vi "HFRR ADV v04 new software.vi"() -> ()   [LabVIEW 2025] (continued)
            n2731 = Search and Replace String(input string=w3755, search string=".duf", replace string=".dgf" ("replace string (\"\")")) -> (result string=→"String Indicator 4":string)  [unwired: 5 in, 3 out]
            n2732 = Match Pattern(string=w3770, regular expression=".dwm") -> (before substring=w3754:string)  [unwired: 1 in, 3 out]
            "String Indicator" <- w3754
            n2733 = Match Pattern(string=w3755, regular expression=".dwm" ("substring (\"\")")) -> (before substring=w3756:string)  [unwired: 1 in, 3 out]
            "String Indicator 3" <- w3756
            n2734 = local write "TITTLE 2"(w3754) -> ()
            n2735 = String To Path(string=w3756) -> (path=w3763:path)
            "path" <- w3763
            n2736 = call <vilib>:"Read Characters From File.vi"("file path (dialog if empty)"=w3763, "start of read offset (chars.:0)"=60 ("start of read offset (chars.: 0)")) -> ("character string"=→"String Indicator 2":string)  [unwired: 4 in, 3 out]
          }
        }
        n2737 = call <vilib>:"Query Available Printers.vi"() -> ("system configured printers"=w3455:string[])  [unwired: 9 in, 2 out]
        "System Configured Printers 2" <- w3455
        n2738 = local read "OK Button 16"() -> (w3452:bool)
        n2739 = case shown="True" "OK Button 16" {
          frame False {
          }
          frame True {
            n2740 = stacked-sequence {
              frame #0 {
                n2741 = local read "Numeric 16"() -> (w3780:i32)
                n2742 = local write "Numeric 10"(w3780) -> ()
              }
              frame #1 {
                n2743 = local read "S.NO"() -> (→"s.NO":string)
                n2744 = local read "String 29"() -> (w3784:string)
                n2745 = String To Path(string=w3784) -> (path=w3783:path)
                n2746 = Open/Create/Replace File "Open File"(file path (use dialog)=w3783) -> (refnum out=w3785:refnum<file>)  [unwired: 5 in, 2 out]
                n2747 = for {
                  N: 16 -> [_]
                  tunnel: w3785 -> [w3792]
                  i -> [w3788]
                  (unwired) TRUE ("line mode (F)")
                  n2748 = Read from Text File "Read File"(file (use dialog)=w3792) -> (text=w3786:string)  [unwired: 3 in, 3 out]
                  n2749 = Match Pattern(string=w3786, regular expression="(") -> (after substring=w3791:string)  [unwired: 1 in, 3 out]
                  n2750 = Match Pattern(string=w3791, regular expression=")") -> (before substring=w3787:string)  [unwired: 1 in, 3 out]
                  n2751 = case shown="1" w3788 {
                    tunnel: w3787 -> [w3793 w3794 _ _ w3795 w3796 w3797 w3799 w3801 w3803 w3805 w3807 w3809 w3811 _]
                    tunnel: w3786 -> [_ _ _ _ _ _ _ _ _ _ _ _ _ _ _]
                    frame 0 {
                      "TITTLE" <- w3793
                    }
                    frame 1 {
                      "Sample ID" <- w3794
                    }
                    frame 2 {
                    }
                    frame 3 {
                    }
                    frame 4 {
                      "Test Date" <- w3795
                    }
                    frame 5 {
                      "Tested by" <- w3796
                    }
                    frame 6 {
                      n2752 = Fract/Exp String To Number(string=w3797) -> (number=→"Humidity before test 2":dbl)  [unwired: 3 in, 1 out]
                    }
                    frame 7 {
                      n2753 = Fract/Exp String To Number(string=w3799) -> (number=→"Temperature before test 2":dbl)  [unwired: 3 in, 1 out]
                    }
                    frame 8 {
                      n2754 = Fract/Exp String To Number(string=w3801) -> (number=→"Humidity after test 2":dbl)  [unwired: 3 in, 1 out]
                    }
                    frame 9 {
                      n2755 = Fract/Exp String To Number(string=w3803) -> (number=→"Temperature after test 2":dbl)  [unwired: 3 in, 1 out]
                    }
                    frame 10 {
                      n2756 = Fract/Exp String To Number(string=w3805) -> (number=→"MWSD 2":dbl)  [unwired: 3 in, 1 out]
                    }
                    frame 11 {
                      n2757 = Fract/Exp String To Number(string=w3807) -> (number=→"AVP 2":dbl)  [unwired: 3 in, 1 out]
                    }
                    frame 12 {
                      n2758 = Fract/Exp String To Number(string=w3809) -> (number=→"HCF 2":dbl)  [unwired: 3 in, 1 out]
                    }
                    frame 13 {
                      n2759 = Fract/Exp String To Number(string=w3811) -> (number=→"WS1.4 2":dbl)  [unwired: 3 in, 1 out]
                    }
                    frame 14, Default {
                    }
                  }
                }
              }
              frame #2 {
              }
            }
            n2760 = local write "OK Button 16"(FALSE ("OK Button 13")) -> ()
          }
        }
        n2761 = Index Array(array=w3455, index="Select Printer 3") -> (element=w3457:string)
        "Selected Printer" <- w3457
        n2762 = case shown="True" w3452 {
          frame False {
          }
          frame True {
            n2763 = flat-sequence {
              frame #0 {
              }
              frame #1 {
                n2764 = Wait (ms)(milliseconds to wait=u32 100) -> ()  [unwired: 1 out]
              }
              frame #2 {
                n2765 = local write "OK Button 16"(FALSE ("Print 3")) -> ()
              }
            }
          }
        }
        n2766 = case shown="True" "Print" {
          tunnel: w3457 -> [_ w3749]
          frame False {
          }
          frame True {
            (unwired) i16 6 ("width (-)")
            (unwired) "TESTED BY : "
            (unwired) "TESTED DATE :"
            (unwired) "SAMPLE ID : "
            (unwired) "SAMPLE DESIGN : "
            w3707 = "\r"
            w3724 = "\r"
            # "add image"
            n2767 = local read "Sample ID"() -> (w3697:string)
            n2768 = local read "Tested by"() -> (w3700:string)
            n2769 = local read "String 34"() -> (w3687:string)
            n2770 = local read "String 45"() -> (w3667:string)
            n2771 = local read "String 35"() -> (w3682:string)
            n2772 = local read "String 37"() -> (w3680:string)
            n2773 = local read "String 32"() -> (w3702:string)
            n2774 = local read "String 36"() -> (w3677:string)
            n2775 = local read "String 31"() -> (w3701:string)
            n2776 = local read "Test Date"() -> (w3698:string)
            n2777 = local read "String 33"() -> (w3703:string)
            n2778 = local read "String 38"() -> (w3673:string)
            n2779 = local read "String 39"() -> (w3670:string)
            n2780 = local write "Print"(FALSE ("Print FF")) -> ()
            n2781 = local read "S 39"() -> (w3685:string)
            n2782 = local read "S 38"() -> (w3692:string)
            n2783 = local read "Temperature before test 2"() -> (w3723:dbl)
            n2784 = local read "Temperature after test 2"() -> (w3713:dbl)
            n2785 = local read "Humidity before test 2"() -> (w3738:dbl)
            n2786 = local read "Humidity after test 2"() -> (w3722:dbl)
            n2787 = local read "MWSD 2"() -> (w3727:dbl)
            n2788 = local read "WS1.4 2"() -> (w3705:dbl)
            n2789 = Concatenate Strings("2)" ("string"), w3687) -> (w3688:string)
            n2790 = Concatenate Strings("3)" ("string"), w3685) -> (w3686:string)
            n2791 = Concatenate Strings("1)" ("string"), w3692) -> (w3691:string)
            n2792 = Concatenate Strings("4)" ("string"), w3682) -> (w3683:string)
            n2793 = Concatenate Strings("5)" ("string"), w3680) -> (w3679:string)
            n2794 = Concatenate Strings("6)" ("string"), w3677) -> (w3676:string)
            n2795 = Concatenate Strings("7)" ("string"), w3673) -> (w3674:string)
            n2796 = Concatenate Strings("8)" ("string"), w3670) -> (w3671:string)
            n2797 = local read "HCF 2"() -> (w3709:dbl)
            n2798 = local read "AVP 2"() -> (w3726:dbl)
            n2799 = local read "s.NO"() -> (w3668:string)
            n2800 = call <vilib>:"New Report.vi"("report type"=enum16{"Standard Report", "HTML"}."Standard Report") -> ("report out"=w3747:refnum<class "NI_report.lvclass">, "error out"=w3746:errorcluster)  [unwired: 13 in]
            n2801 = local read "TITTLE"() -> (w3699:string)
            n2802 = Concatenate Strings(w3724, w3667, w3668, w3724, w3702, w3697, w3724, w3701, w3698, w3724, w3703, w3700, w3724) -> (w3717:string)
            "test by" <- w3717
            n2803 = Number To Fractional String(number=w3723, width (-)=i16 6, precision (6)=i16 2) -> (F-format string=w3712:string)  [unwired: 1 in]
            n2804 = Number To Fractional String(number=w3722, width (-)=i16 6, precision (6)=i16 2) -> (F-format string=w3725:string)  [unwired: 1 in]
            n2805 = Number To Fractional String(number=w3738, width (-)=i16 6, precision (6)=i16 2) -> (F-format string=w3743:string)  [unwired: 1 in]
            n2806 = Number To Fractional String(number=w3727, width (-)=i16 6, precision (6)=i16 2) -> (F-format string=w3729:string)  [unwired: 1 in]
            n2807 = Number To Fractional String(number=w3713, width (-)=i16 6, precision (6)=i16 2) -> (F-format string=w3714:string)  [unwired: 1 in]
            n2808 = Number To Fractional String(number=w3726, width (-)=i16 6, precision (6)=i16 2) -> (F-format string=w3728:string)  [unwired: 1 in]
            n2809 = Number To Fractional String(number=w3709, width (-)=i16 6, precision (6)=i16 2) -> (F-format string=w3708:string)  [unwired: 1 in]
            n2810 = Number To Fractional String(number=w3705, precision (6)=i16 2) -> (F-format string=w3704:string)  [unwired: 2 in]
            n2811 = call-dynamic "Set Report Header Text.vi"("report in"=w3747, "center header text"=w3699, "error in (no error)"=w3746) -> ("report out"=w3718:refnum<class "NI_report.lvclass">, "error out"=w3719:errorcluster)  [unwired: 11 in]
            n2812 = Concatenate Strings(w3707, w3691, w3743, w3707, w3688, w3712, w3707, w3686, w3725, w3707, w3683, w3714, w3707, w3679, w3729, w3707, w3676, w3728, w3707, w3674, w3708, w3707, w3671, w3704) -> (w3695:string)
            "export 2" <- w3695
            n2813 = call-poly <vilib>:"Append Report Text.vi"("report in"=w3718, "text"=w3717, "error in (no error)"=w3719) -> ("report out"=w3721:refnum<class "NI_report.lvclass">, "error out"=w3720:errorcluster)  [unwired: 9 in, 2 out]
            n2814 = local read "test by"() -> (w3694:string)
            n2815 = local read "TITTLE"() -> (w3696:string)
            n2816 = call-poly <vilib>:"Append Report Text.vi"("report in"=w3721, "error in (no error)"=w3720) -> ("report out"=w3742:refnum<class "NI_report.lvclass">, "error out"=w3740:errorcluster)  [unwired: 10 in, 2 out]
            n2817 = Concatenate Strings(w3696, w3695, w3694) -> (→"output":string)
            n2818 = call-poly <vilib>:"Append Report Text.vi"("report in"=w3742, "text"=w3695, "error in (no error)"=w3740) -> ("report out"=w3741:refnum<class "NI_report.lvclass">, "error out"=w3739:errorcluster)  [unwired: 9 in, 2 out]
            n2819 = call-dynamic "Print Report.vi"("report in"=w3741, "printer name (default)"=w3749, "error in (no error)"=w3739) -> ("report out"=w3751:refnum<class "NI_report.lvclass">, "error out"=w3752:errorcluster)  [unwired: 11 in]
            n2820 = call-dynamic "Dispose Report.vi"("report in"=w3751, "error in (no error)"=w3752) -> ()  [unwired: 13 in, 1 out]
          }
        }
        n2821 = case shown="True" "Print 2" {
          frame False {
          }
          frame True {
            n2822 = flat-sequence {
              frame #0 {
                n2823 = local read "s.NO"() -> (→"s.NO 2":string)
                n2824 = Wait (ms)(milliseconds to wait=u32 20) -> ()  [unwired: 1 out]
                n2825 = local read "Sample ID  3"() -> (→"Sample ID  6":string)
                n2826 = local read "Sample ID  4"() -> (→"Sample ID  7":string)
                n2827 = local read "Sample ID"() -> (→"Sample ID  2":string)
                n2828 = local read "Tested by"() -> (→"Tested by 2":string)
                n2829 = local read "Test Date"() -> (→"Test Date 2":string)
                n2830 = local read "Humidity after test 3"() -> (→"Humidity after test 4":dbl)
                n2831 = local read "Ref A Test Date :"() -> (→"TITTLE 4":string)
                n2832 = local read "Temperature before test 3"() -> (w3574:dbl)
                n2833 = local read "Temperature before test 3"() -> (→"Temperature after test 5":dbl)
                n2834 = local read "Temperature after test 3"() -> (→"Temperature after test 4":dbl)
                n2835 = local read "Humidity before test 3"() -> (→"Humidity before test 4":dbl)
                n2836 = local write "Temperature before test 3"(w3574) -> ()
                n2837 = local read "image data"() -> (w3565:T11)
                n2838 = String To Path(string="C:\\LAB-IQ\\im\\Temp_resized.jpg") -> (path=w3566:path)
                "path 2" <- w3566
                n2839 = call <vilib>:"Write JPEG File.vi"("image data"=w3565, "path to JPEG file"=w3566) -> ()  [unwired: 8 in, 2 out]
                "Ref A Test Date :" <- "Ref A Test Date :"
                "Ref B Test Date :" <- "Ref B Test Date :"
                "Ref B Scar Value :" <- "Ref B Scar Value :"
                "Ref A Scar Value :" <- "Ref A Scar Value :"
              }
              frame #1 {
                (unwired) HTML_Report_Image_Alignment."MIDDLE" ("alignment (default)")
                w3602 = u16 0 items=["portrait", "landscape"] ("orientation (portrait)")
                (unwired) HTML_Report_Image_Alignment."ABSMIDDLE" ("alignment (default)")
                (unwired) "TESTED BY : "
                (unwired) "TESTED DATE :"
                (unwired) "SAMPLE ID : "
                (unwired) "SAMPLE DESIGN : "
                w3635 = "\r"
                # "add image"
                n2840 = Wait (ms)(milliseconds to wait=u32 20) -> ()  [unwired: 1 out]
                n2841 = local read "Sample ID  2"() -> (w3628:string)
                n2842 = local read "Wear Scar X"() -> (w3600:dbl)
                "Length ( microns ) 2" <- w3600
                n2843 = local read "Wear Scar Y"() -> (w3599:dbl)
                "Wear Scar Y ( microns ) :" <- w3599
                n2844 = local read "Test Date 2"() -> (w3629:string)
                n2845 = local read "Tested by 2"() -> (w3630:string)
                n2846 = local read "String 46"() -> (w3626:string)
                n2847 = local read "String 48"() -> (w3632:string)
                n2848 = local read "String 47"() -> (w3631:string)
                n2849 = local read "String 49"() -> (w3633:string)
                n2850 = local read "String 10"() -> (w3586:string)
                n2851 = local read "s.NO 2"() -> (w3627:string)
                n2852 = Add(x=w3600, y=w3599) -> (x+y=w3598:dbl)
                n2853 = call <vilib>:"New Report.vi"("report type"=enum16{"Standard Report", "HTML"}."HTML") -> ("report out"=w3606:refnum<class "NI_report.lvclass">, "error out"=w3604:errorcluster)  [unwired: 13 in]
                n2854 = Concatenate Strings(w3635, w3626, w3627, w3635, w3632, w3628, w3635, w3631, w3629, w3635, w3633, w3630, w3635) -> (→"test by 2":string)
                n2855 = Concatenate Strings("C:\\LAB-IQ\\Data\\" ("string"), w3586, ".jpg" ("string")) -> ()  [unwired: 1 out]
                n2856 = Divide(x=w3598, y=2.0) -> (x/y=→"Mean Wear ( microns) :":dbl)
                n2857 = call-dynamic "Set Report Orientation.vi"("report in"=w3606, "orientation (portrait)"=w3602, "error in (no error)"=w3604) -> ("report out"=w3605:refnum<class "NI_report.lvclass">, "error out"=w3603:errorcluster)  [unwired: 11 in]
                n2858 = for {
                  N: 5 -> [_]
                  tunnel: w3605 -> [w3656]
                  tunnel: [w3655] -> w3584
                  tunnel: w3603 -> [w3654]
                  tunnel: [w3653] -> w3583
                  n2859 = call-dynamic "Set Report Tab Width.vi"("report in"=w3656, "error in (no error)"=w3654) -> ("report out"=w3655:refnum<class "NI_report.lvclass">, "error out"=w3653:errorcluster)  [unwired: 12 in]
                }
                n2860 = local read "TITTLE"() -> (w3601:string)
                n2861 = call-dynamic "Set Report Header Text.vi"("report in"=w3584, "center header text"=w3601, "error in (no error)"=w3583) -> ("report out"=w3622:refnum<class "NI_report.lvclass">, "error out"=w3621:errorcluster)  [unwired: 11 in]
                n2862 = for {
                  N: 1 -> [_]
                  tunnel: [w3660] -> w3608
                  tunnel: [w3659] -> w3607
                  tunnel: w3622 -> [w3658]
                  tunnel: w3621 -> [w3657]
                  n2863 = call-dynamic "New Report Line.vi"("report in"=w3658, "error in (no error)"=w3657) -> ("report out"=w3660:refnum<class "NI_report.lvclass">, "error out"=w3659:errorcluster)  [unwired: 12 in]
                }
                n2864 = for {
                  N: 2 -> [_]
                  tunnel: [w3652] -> w3614
                  tunnel: [w3651] -> w3613
                  tunnel: w3608 -> [w3650]
                  tunnel: w3607 -> [w3649]
                  n2865 = call-dynamic "New Report Line.vi"("report in"=w3650, "error in (no error)"=w3649) -> ("report out"=w3652:refnum<class "NI_report.lvclass">, "error out"=w3651:errorcluster)  [unwired: 12 in]
                }
                n2866 = for {
                  N: 25 -> [_]
                  tunnel: w3614 -> [w3648]
                  tunnel: w3613 -> [w3646]
                  tunnel: [w3647] -> w3617
                  tunnel: [w3645] -> w3616
                  n2867 = call-dynamic "Set Report Tab Width.vi"("report in"=w3648, "error in (no error)"=w3646) -> ("report out"=w3647:refnum<class "NI_report.lvclass">, "error out"=w3645:errorcluster)  [unwired: 12 in]
                }
                n2868 = control-ref of="Tab Control 9"() -> (w3612:refnum<vi>)
                n2869 = call-dynamic "Append Control Image to Report.vi"("report in"=w3617, "alignment (default)"=HTML_Report_Image_Alignment."ABSMIDDLE", "ctrl reference"=w3612, "error in (no error)"=w3616) -> ("report out"=w3611:refnum<class "NI_report.lvclass">, "error out"=w3610:errorcluster)  [unwired: 8 in, 2 out]
                n2870 = for {
                  N: 3 -> [_]
                  tunnel: [w3644] -> w3595
                  tunnel: [w3643] -> w3594
                  tunnel: w3611 -> [w3642]
                  tunnel: w3610 -> [w3641]
                  n2871 = call-dynamic "New Report Line.vi"("report in"=w3642, "error in (no error)"=w3641) -> ("report out"=w3644:refnum<class "NI_report.lvclass">, "error out"=w3643:errorcluster)  [unwired: 12 in]
                }
                n2872 = for {
                  N: 100 -> [_]
                  tunnel: w3595 -> [w3640]
                  tunnel: w3594 -> [w3638]
                  tunnel: [w3639] -> w3591
                  tunnel: [w3637] -> w3589
                  n2873 = call-dynamic "Set Report Tab Width.vi"("report in"=w3640, "error in (no error)"=w3638) -> ("report out"=w3639:refnum<class "NI_report.lvclass">, "error out"=w3637:errorcluster)  [unwired: 12 in]
                }
                n2874 = String To Path(string="C:\\LAB-IQ\\im\\Temp_resized.jpg") -> (path=w3581:path)
                n2875 = call-poly <vilib>:"Append Image to Report.vi"("report in"=w3591, "path or URL of image"=w3581, "error in (no error)"=w3589) -> ("report out"=w3590:refnum<class "NI_report.lvclass">, "error out"=w3588:errorcluster)  [unwired: 9 in, 2 out]
                n2876 = call-poly <vilib>:"Open HTML Report in Browser.vi"("report in"=w3590, "error in (no error)"=w3588) -> ("report out"=w3625:refnum<class "NI_report.lvclass">, "error out"=w3624:errorcluster)  [unwired: 11 in, 1 out]
                n2877 = call-dynamic "Dispose Report.vi"("report in"=w3625, "error in (no error)"=w3624) -> ()  [unwired: 13 in, 1 out]
              }
              frame #2 {
              }
              frame #3 {
                n2878 = disable-structure shown="Disabled" {
                  frame Disabled {
                    n2879 = local read "String 10"() -> (w3665:string)
                    n2880 = Concatenate Strings("C:\\LAB-IQ-NXT\\Data\\" ("string"), w3665, ".jpg" ("string")) -> (w3663:string)
                    n2881 = String To Path(string=w3663) -> (path=w3662:path)
                    n2882 = Delete(path (use dialog)=w3662) -> ()  [unwired: 4 in, 3 out]
                  }
                  frame Enabled {
                  }
                }
                n2883 = local write "Print 2"(FALSE ("Print")) -> ()
              }
            }
          }
        }
      }
    }
    n2884 = property on="SetTemp" class="DigNum (strict)"("Disabled"=w1621) -> ()  [unwired: 2 in, 2 out]
    n2885 = Multiply(x=w1611, y=w1613) -> (x*y=w1612:dbl)
    n2886 = local read "MWSD"() -> (w1610:dbl)
    n2887 = Add(x=w1612, y=w1610) -> (x+y=→"WS1.4":dbl)
    n2888 = Wait (ms)(milliseconds to wait=u32 50) -> ()  [unwired: 1 out]
    n2889 = Wait (ms)(milliseconds to wait=u32 50) -> ()  [unwired: 1 out]
    n2890 = local read "Quit"() -> (w1609:bool)
  }
  n2891 = VISA Close(VISA resource name=w52, error in (no error)=w51) -> (error out=w49:errorcluster)
  n2892 = call <vilib>:"Clear Errors.vi"("error in (no error)"=w49) -> ()  [unwired: 5 in, 2 out]
  n2893 = VISA Close(VISA resource name=w37, error in (no error)=w36) -> ()  [unwired: 1 out]
  n2894 = while {
    tunnel: [w3824] -> w46
    shift-right: [w3817] -> _
    shift-left: 0.0 -> [w3820]
    shift-right: [w3816] -> _
    shift-left: 0.0 -> [w3819]
    shift-right: [w3815] -> _
    shift-left: 400.0 ("vc_cmd") -> [w3818]
    stop <- w3824 stop-if-true
    # "PID LOGIC"
    n2895 = local read "RUN"() -> (w3822:bool)
    n2896 = local read "Auto Start Test"() -> (w3821:bool)
    n2897 = local read "START TEMP"() -> (w3813:bool)
    n2898 = Or(x=w3822, y=w3821) -> (x .or. y?=w3823:bool)
    n2899 = And(x=w3823, y=w3813) -> (x .and. y?=w3814:bool)
    n2900 = Wait (ms)(milliseconds to wait=u32 20) -> ()  [unwired: 1 out]
    n2901 = case shown="True" w3814 {
      tunnel: [400.0 ("out_vc_cmd") w3844] -> w3815
      tunnel: [w3827 w3846] -> w3816
      tunnel: [w3827 w3845] -> w3817
      tunnel: w3820 -> [_ w3834]
      tunnel: w3819 -> [_ w3833]
      tunnel: w3818 -> [_ w3832]
      frame False {
        w3827 = 0.0 ("error_out")
      }
      frame True {
        n2902 = local read "Set Strk"() -> (w3829:dbl)
        n2903 = local read "measured_stroke"() -> (w3835:dbl)
        n2904 = Add(x=w3829, y="Add up Stroke") -> (x+y=w3830:dbl)
        n2905 = formula code="// Zero-Hardcode Explicit Positional-Form PID Engine\n// Inputs: target_stroke, measured_stroke, dt, prev_error, integral_accumulator_in, prev_vc_cmd\n//         kp, ki, kd, max_step_change, max_amplitude, min_amplitude, startup_cmd\n// Outputs: vc_cmd, error_out, out_error, integral_accumulator_out, out_vc_cmd\n\n// 1. Calculate Tracking Error\nfloat current_error = target_stroke - measured_stroke;\nerror_out = current_error;\n\n// 2. Compute Proportional Term\nfloat p_term = kp * current_error;\n\n// 3. Compute Derivative Term\nfloat d_term = 0.0;\nif (dt > 0.0) {\n    d_term = kd * ((current_error - prev_error) / dt);\n}\n\n// 4. Update and Accumulate Integral Term\nfloat current_integral = integral_accumulator_in + (current_error * dt);\nfloat i_term = ki * current_integral;\n\n// 5. Calculate Ideal Target Command\nfloat ideal_command = startup_cmd + p_term + i_term + d_term;\n\n// 6. Anti-Windup Protection (Back-calculation method)\nif (ideal_command > max_amplitude) {\n    float excess = ideal_command - max_amplitude;\n    if (ki > 0.0) {\n        current_integral -= excess / ki;\n    }\n    ideal_command = max_amplitude;\n} else if (ideal_command < min_amplitude) {\n    float excess = ideal_command - min_amplitude;\n    if (ki > 0.0) {\n        current_integral -= excess / ki;\n    }\n    ideal_command = min_amplitude;\n}\n\n// 7. Apply Loop Rate Limiting (Protects voice coil from large voltage steps)\nfloat raw_adjustment = ideal_command - prev_vc_cmd;\n\nif (raw_adjustment > max_step_change) {\n    raw_adjustment = max_step_change;\n} else if (raw_adjustment < -max_step_change) {\n    raw_adjustment = -max_step_change;\n}\n\nfloat next_vc_cmd = prev_vc_cmd + raw_adjustment;\n\n// Final Output Safety Safeguard Clamping\nif (next_vc_cmd > max_amplitude) {\n    next_vc_cmd = max_amplitude;\n} else if (next_vc_cmd < min_amplitude) {\n    next_vc_cmd = min_amplitude;\n}\n\n// 8. Map to Shift Registers for memory persistence\nvc_cmd = next_vc_cmd;\nout_error = current_error;                     \nintegral_accumulator_out = current_integral;  \nout_vc_cmd = next_vc_cmd;"("target_stroke"=w3830, "measured_stroke"=w3835, "dt"="dt", "integral_accumulator_in"=w3833, "prev_error"=w3834, "prev_vc_cmd"=w3832, "kp"="kp", "ki"="ki", "kd"="kd", "max_step_change"="max_step_change", "max_amplitude"="max_amplitude", "min_amplitude"="min_amplitude", "startup_cmd"="startup_cmd") -> ("vc_cmd"=w3850:dbl, "out_error"=w3845:dbl, "integral_accumulator_out"=w3846:dbl, "out_vc_cmd"=w3844:dbl)  [unwired: 1 out]
        "output Vpp" <- w3850
        n2906 = Number To Fractional String(number=w3850, precision (6)=i16 1) -> (F-format string=w3848:string)  [unwired: 2 in]
        n2907 = Concatenate Strings("DAC;" ("string"), w3848) -> (w3831:string)
        n2908 = local write "Command"(w3831) -> ()
        "prev_error" <- w3834
        "integral_accumulator_in" <- w3833
        "prev_vc_cmd" <- w3832
      }
    }
    n2909 = local read "Quit"() -> (w3824:bool)
  }
  n2910 = Or(x=w42, y=w41) -> (x .or. y?=w43:bool)
  n2911 = Or(x=w39, y=w43) -> (x .or. y?=w48:bool)
  n2912 = control-ref of="new picture"() -> ()  [unwired: 1 out]
  n2913 = Or(x=w54, y=w48) -> (x .or. y?=w45:bool)
  n2914 = Or(x=w45, y=w46) -> (x .or. y?=w40:bool)
  n2915 = while {
    tunnel: [w3851] -> w53
    i -> [w3858]
    stop <- w3851 stop-if-true
    n2916 = local read "Quit"() -> (w3851:bool)
    n2917 = Equal To 0?(x=w3858) -> (x = 0?=w3856:bool)
    n2918 = call "Elapsed Time3"("Time Target (s)"=45.0, "Auto Reset"=TRUE) -> ("Time has Elapsed"=w3855:bool)  [unwired: 10 in, 7 out]
    n2919 = Wait (ms)(milliseconds to wait=u32 50) -> ()  [unwired: 1 out]
    n2920 = Or(x=w3855, y=w3856) -> (x .or. y?=w3857:bool)
    n2921 = case shown="True" w3857 {
      frame False {
      }
      frame True {
        n2922 = call <vilib>:"System Exec.vi"("run minimized? (F)"=TRUE, "error in (no error)"="error in (no error)", "command line"="powercfg.exe -change -monitor-timeout-ac 0") -> ("error out"=w3869:errorcluster)  [unwired: 5 in, 3 out]
        n2923 = call <vilib>:"System Exec.vi"("run minimized? (F)"=TRUE, "error in (no error)"=w3869, "command line"="powercfg.exe -change -disk-timeout-ac 0") -> ("error out"=w3868:errorcluster)  [unwired: 5 in, 3 out]
        n2924 = call <vilib>:"System Exec.vi"("run minimized? (F)"=TRUE, "error in (no error)"=w3868, "command line"="powercfg.exe -change -standby-timeout-ac 0") -> ("error out"=w3867:errorcluster)  [unwired: 5 in, 3 out]
        n2925 = call <vilib>:"System Exec.vi"("run minimized? (F)"=TRUE, "error in (no error)"=w3867, "command line"="powercfg.exe -change -hibernate-timeout-ac 0") -> ("error out"=w3866:errorcluster)  [unwired: 5 in, 3 out]
        n2926 = call <vilib>:"Simple Error Handler.vi"("error in (no error)"=w3866) -> ("error out"=w3872:errorcluster)  [unwired: 4 in, 4 out]
        n2927 = call <vilib>:"Clear Errors.vi"("error in (no error)"=w3872) -> ("error out"=→"error out":errorcluster)  [unwired: 5 in, 1 out]
      }
    }
  }
  n2928 = Compound Arithmetic op=OR(w56, w40, w53) -> (w55:bool)
  n2929 = flat-sequence {
    tunnel: w55 -> [_]
    tunnel: [w3874] -> w17
    tunnel: w17 -> [_]
    frame #0 {
      n2930 = call "CLOSE CONNECTION.vi"() -> ("error out"=w3874:errorcluster)  [unwired: 11 in]
    }
    frame #1 {
      n2931 = Quit LabVIEW(quit? (T)=TRUE) -> ()
      n2932 = local write "Quit"(FALSE ("EXIT")) -> ()
    }
  }
  n2933 = property on="Heater Button" class="Bool (strict)"("Visible"=TRUE) -> ()  [unwired: 2 in, 2 out]
  n2934 = disable-structure shown="Disabled" {
    disable-tunnel: _ -> [w3880 _]
    disable-tunnel: _ -> [w3877 _]
    disable-tunnel: _ -> [w3878 _]
    frame Disabled {
      n2935 = disable-structure shown="Disabled" {
        disable-tunnel: [w3887 _] -> w3879
        frame Disabled {
          n2936 = while {
            shift-right: [w3929] -> w3885
            shift-left: errorcluster {"status"=TRUE, "code"=0, "source"="Init"} ("error out") -> [w3894]
            shift-right: [w3928] -> w3884
            shift-left: _ -> [w3895]
            shift-right: [w3927] -> _
            shift-left: "" -> [w3926]
            tunnel: [w3888] -> w3887
            shift-right: ["Set Rh"] -> _
            shift-left: 0.0 ("Set Rh") -> [w3920]
            tunnel: [w3897] -> _
            i -> [w3897]
            stop <- w3888 stop-if-true
            n2937 = flat-sequence {
              tunnel: w3894 -> [w3932]
              tunnel: [w3932] -> w3893
              frame #0 {
                n2938 = Wait (ms)(milliseconds to wait=u32 200) -> ()  [unwired: 1 out]
              }
            }
            n2939 = local read "Com Port 3"() -> (w3896:refnum<visa-resource-name>)
            n2940 = local read "Humidity Str Rec"() -> (w3898:string)
            n2941 = Not Equal?(x="Set Rh", y=w3920) -> (x != y?=w3925:bool)
            n2942 = Number To Decimal String(number="Set Rh") -> (decimal integer string=w3923:string)  [unwired: 1 in]
            n2943 = Not Equal?(x=w3896, y=w3895) -> (x != y?=w3891:bool)
            n2944 = Concatenate Strings("#setPoint00" ("string"), w3923) -> (w3924:string)
            n2945 = case shown="False" w3925 {
              tunnel: w3924 -> [_ w3944]
              frame False {
                n2946 = local read "Humidity"() -> (w3941:bool)
                n2947 = case shown="True" w3941 {
                  frame False {
                    n2948 = local write "Humidity Str Send"("stop" ("Humidity Str Send")) -> ()
                  }
                  frame True {
                    n2949 = local write "Humidity Str Send"("start" ("Humidity Str Send")) -> ()
                  }
                }
              }
              frame True {
                n2950 = local write "Humidity Str Send"(w3944) -> ()
              }
            }
            n2951 = Or(x=w3891) -> (y=w3889:bool, x .or. y?=w3890:bool)
            n2952 = String Subset(string=w3898, offset (0)=7) -> (substring=w3913:string)  [unwired: 1 in]
            n2953 = Match Pattern(string=w3898, regular expression="?") -> (offset past match=w3916:i32)  [unwired: 1 in, 3 out]
            n2954 = Match Pattern(string=w3898, regular expression="v") -> (offset past match=w3919:i32)  [unwired: 1 in, 3 out]
            n2955 = case shown="True" w3890 {
              tunnel: w3893 -> [w3930 _]
              tunnel: [w3930 errorcluster {"status"=TRUE, "code"=0, "source"="Init"} ("error out")] -> w3892
              frame False {
              }
              frame True {
              }
            }
            n2956 = Equal?(x=w3916, y=-1) -> (x = y?=w3900:bool)
            n2957 = Match Pattern(string=w3913, regular expression="g") -> (after substring=w3914:string, offset past match=w3905:i32)  [unwired: 1 in, 2 out]
            n2958 = Match Pattern(string=w3913, regular expression="y") -> (after substring=w3912:string, offset past match=w3906:i32)  [unwired: 1 in, 2 out]
            n2959 = Greater?(x=w3906, y=w3905) -> (0:w3911:bool)
            n2960 = Greater Or Equal To 0?(x=w3906) -> (x >= 0?=w3903:bool)
            n2961 = Greater Or Equal To 0?(x=w3905) -> (x >= 0?=w3904:bool)
            n2962 = Or(x=w3903, y=w3904) -> (x .or. y?=w3902:bool)
            n2963 = Greater Or Equal To 0?(x=w3919) -> (x >= 0?=w3901:bool)
            n2964 = Select(t=w3912, s=w3911, f=w3914) -> (s? t:f=w3907:string)
            n2965 = case shown="Error" w3892 {
              selector: w3892 -> [w3957 w4003]
              tunnel: [w3955 w3996] -> w3929
              tunnel: w3895 -> [w3958 w4002]
              tunnel: [w3956 w4005] -> w3928
              tunnel: w3926 -> [w3945 w4004]
              tunnel: [w3952 w4004] -> w3927
              frame No Error {
                n2966 = call "Elapsed Time7"() -> ("Time has Elapsed"=w3951:bool)  [unwired: 12 in, 7 out]
                n2967 = Not Equal?(x="Humidity Str Send", y=w3945) -> (x != y?=w3947:bool)
                n2968 = Or(x=w3947, y=w3951) -> (x .or. y?=w3950:bool)
                n2969 = Select(t="Humidity Str Send", s=w3947, f="vals" ("regular expression")) -> (s? t:f=w3946:string)
                n2970 = Or(x=w3950, y="Send") -> (x .or. y?=w3954:bool)
                n2971 = case shown="True" w3954 {
                  tunnel: [w3961 w3966] -> w3955
                  tunnel: w3958 -> [w3960 w3974]
                  tunnel: w3957 -> [w3961 w3973]
                  tunnel: [w3960 w3967] -> w3956
                  tunnel: w3946 -> [_ w3972]
                  tunnel: [w3959 w3963] -> w3952
                  tunnel: "Humidity Str Send" -> [_ w3964]
                  tunnel: w3947 -> [_ w3965]
                  tunnel: w3945 -> [w3959 w3962]
                  frame False {
                  }
                  frame True {
                    n2972 = flat-sequence {
                      tunnel: w3974 -> [w3982]
                      tunnel: w3973 -> [w3981]
                      tunnel: w3972 -> [w3978]
                      tunnel: [w3980] -> w3971
                      tunnel: [w3979] -> w3970
                      tunnel: w3971 -> [w3985]
                      tunnel: w3970 -> [w3984]
                      tunnel: [w3985] -> w3969
                      tunnel: [w3984] -> w3968
                      tunnel: w3969 -> [w3992]
                      tunnel: w3968 -> [w3991]
                      tunnel: [w3990] -> w3967
                      tunnel: [w3989] -> w3966
                      frame #0 {
                        n2973 = local write "Ser Led"(TRUE ("Boolean 4")) -> ()
                        n2974 = Concatenate Strings(w3978, "\r") -> (w3977:string)
                        n2975 = VISA Write(VISA resource name=w3982, write buffer=w3977, error in (no error)=w3981) -> (VISA resource name out=w3980:refnum<visa-resource-name>, error out=w3979:errorcluster)  [unwired: 1 out]
                      }
                      frame #1 {
                        n2976 = Wait (ms)(milliseconds to wait="wait") -> ()  [unwired: 1 out]
                      }
                      frame #2 {
                        w3987 = FALSE ("Send")
                        n2977 = property class="Instr"(reference=w3992, error in=w3991) -> (reference out=w3993:refnum<visa-resource-name>, error out=w3994:errorcluster, "Serial Settings:Number of Bytes at Serial Port"=w3986:u32)
                        n2978 = local write "Send"(w3987) -> ()
                        n2979 = local write "Ser Led"(w3987) -> ()
                        n2980 = VISA Read(VISA resource name=w3993, byte count=w3986, error in (no error)=w3994) -> (VISA resource name out=w3990:refnum<visa-resource-name>, read buffer=→"Humidity Str Rec":string, error out=w3989:errorcluster)  [unwired: 1 out]
                      }
                    }
                    n2981 = Select(t=w3964, s=w3965, f=w3962) -> (s? t:f=w3963:string)
                  }
                }
              }
              frame Error {
                w4010 = u16 0 items=["None"=0, "XON/XOFF"=1, "RTS/CTS"=2, "DTR/DSR"=4] ("flow control")
                w4006 = u16 0 items=["None", "Odd", "Even", "Mark", "Space"] ("parity")
                w4009 = u16 10 items=["1.0"=10, "1.5"=15, "2.0"=20] ("stop bits")
                n2982 = VISA Close(VISA resource name=w4002, error in (no error)=w4003) -> (error out=w4001:errorcluster)
                n2983 = local write "humid"("" ("humid")) -> ()
                n2984 = local write "Humidity Str Rec"("" ("Humidity Str Rec")) -> ()
                n2985 = call <vilib>:"Clear Errors.vi"("error in (no error)"=w4001) -> ("error out"=w4000:errorcluster)  [unwired: 5 in, 1 out]
                n2986 = local read "Com Port 3"() -> (w3999:refnum<visa-resource-name>)
                n2987 = call-poly "VISA Configure Serial Port"("VISA resource name"=w3999, "timeout (10sec)"=u32 1000, "termination char\n(0xA = '\\n' = LF)"=u8 10 ("termination char\n(0xA = '\\n' = LF)"), "Enable Termination\nChar (T)"=FALSE ("Enable Termination Char (T)"), "data bits (8)"=u16 8 ("data bits"), "parity (0:none)"=w4006, "error in (no error)"=w4000, "stop bits (10: 1 bit)"=w4009, "flow control (0:none)"=w4010) -> ("VISA resource name out"=w4005:refnum<visa-resource-name>, "baud rate (9600)"=w3997:u32, "error out"=w3996:errorcluster)  [unwired: 4 in]
              }
            }
            n2988 = Compound Arithmetic op=AND(w3901, w3900, w3902) -> (w3899:bool)
            n2989 = case shown="True" w3899 {
              tunnel: w3898 -> [_ _]
              tunnel: w3907 -> [_ w3937]
              frame False {
              }
              frame True {
                w3935 = " " ("regular expression")
                n2990 = Match Pattern(string=w3937, regular expression=" ") -> (after substring=w3939:string)  [unwired: 1 in, 3 out]
                n2991 = Match Pattern(string=w3939, regular expression=w3935) -> (before substring=→"humid":string, after substring=w3936:string)  [unwired: 1 in, 2 out]
                n2992 = Match Pattern(string=w3936, regular expression=w3935) -> (before substring=→"temp_@Rh sensor":string)  [unwired: 1 in, 3 out]
              }
            }
            n2993 = local read "Quit"() -> (w3888:bool)
          }
          n2994 = VISA Close(VISA resource name=w3884, error in (no error)=w3885) -> (error out=w3881:errorcluster)
          n2995 = call <vilib>:"Clear Errors.vi"("error in (no error)"=w3881) -> ()  [unwired: 5 in, 2 out]
        }
        frame Enabled {
        }
      }
    }
    frame Enabled {
    }
  }
  n2996 = while {
    tunnel: [w4017] -> _
    i -> [w4017]
    stop <- w4013 stop-if-true
    # "Langauage selection"
    n2997 = Equal?(x="Lan flag", y=22.0) -> ()  [unwired: 1 out]
    n2998 = disable-structure shown="Disabled" {
      frame Disabled {
        n2999 = stacked-sequence {
          frame #0 {
            n3000 = case shown="\"Russian\"" "Language Selection" {
              tunnel: [0 1] -> w4019
              frame "English", Default {
              }
              frame "Russian" {
              }
            }
            n3001 = for {
              N: 130 -> [_]
              tunnel: "Table" -> [w4028]
              tunnel: w4019 -> [w4027]
              i -> [w4026]
              n3002 = Index Array(array=w4028, index (row)=w4026, index (col)=w4027) -> (element=w4025:string)
              n3003 = case shown="123" w4026 {
                tunnel: w4025 -> [w4029 w4030 _ w4031 w4032 w4033 w4034 w4035 w4036 w4037 w4038 w4039 w4040 w4041 w4042 w4043 w4044 w4045 w4046 w4047 w4048 w4049 w4050 w4051 w4052 w4053 w4054 w4055 w4056 _ _ w4057 w4058 w4059 w4060 w4061 w4062 w4071 w4078 w4085 w4092 w4096 w4099 w4102 w4104 w4106 w4107 w4108 w4109 w4110 w4111 w4112 w4113 w4114 w4115 w4116 w4117 w4118 w4119 w4120 w4121 w4122 w4123 w4124 w4125 w4126 w4127 w4128 w4129 w4130 w4131 w4132 w4133 w4134 w4135 w4136 w4137 w4138 w4139 w4140 w4141 w4142 w4143 w4144 w4145 w4146 w4147 w4148 w4149 w4150 w4151 w4152 w4153 w4154 w4155 w4156 w4157 w4158 w4159 w4160 w4161 w4162 w4163 w4164 w4165 _ w4166 w4167 w4168 w4169 w4170 w4171 w4172 w4173 w4174 w4175 w4176 w4177 w4178 _ w4179 w4180 w4181 w4182 w4183 w4184 _]
                frame 0 {
                  n3004 = local write "S"(w4029) -> ()
                }
                frame 1 {
                  n3005 = local write "S 2"(w4030) -> ()
                }
                frame 2 {
                }
                frame 3 {
                  n3006 = local write "S 4"(w4031) -> ()
                }
                frame 4 {
                  n3007 = property on="FILE" class="Str"("Caption.Text"=w4032) -> ()  [unwired: 2 in, 2 out]
                }
                frame 5 {
                  n3008 = property on="Fuel Discription :" class="Str"("Caption.Text"=w4033) -> ()  [unwired: 2 in, 2 out]
                }
                frame 6 {
                  n3009 = property on="Remarks :" class="Str"("Caption.Text"=w4034) -> ()  [unwired: 2 in, 2 out]
                }
                frame 7 {
                  n3010 = property on="Save & Continue" class="Bool (strict)"("Boolean Text.Text"=w4035) -> ()  [unwired: 2 in, 2 out]
                }
                frame 8 {
                }
                frame 9 {
                  n3011 = property on="Set Hz" class="DigNum (strict)"("Caption.Text"=w4037) -> ()  [unwired: 2 in, 2 out]
                }
                frame 10 {
                  "String 3" <- w4038
                }
                frame 11 {
                  n3012 = property on="NORMAL LOAD" class="DigNum (strict)"("Caption.Text"=w4039) -> ()  [unwired: 2 in, 2 out]
                }
                frame 12 {
                  "String 5" <- w4040
                }
                frame 13 {
                  n3013 = property on="Set Temp" class="DigNum (strict)"("Caption.Text"=w4041) -> ()  [unwired: 2 in, 2 out]
                }
                frame 14 {
                  n3014 = local write "S 15"(w4042) -> ()
                }
                frame 15 {
                  n3015 = property on="Set Rh" class="DigNum (strict)"("Caption.Text"=w4043) -> ()  [unwired: 2 in, 2 out]
                }
                frame 16 {
                  "String 13" <- w4044
                  "String 26" <- w4044
                }
                frame 17 {
                  n3016 = local write "S 18"(w4045) -> ()
                }
                frame 18 {
                  "String 17" <- w4046
                }
                frame 19 {
                  n3017 = property on="test time" class="DigNum (strict)"("Caption.Text"=w4047) -> ()  [unwired: 2 in, 2 out]
                }
                frame 20 {
                  "String 18" <- w4048
                  "String 22" <- w4048
                }
                frame 21 {
                  n3018 = property on="Elapsed time" class="DigNum (strict)"("Caption.Text"=w4049) -> ()  [unwired: 2 in, 2 out]
                }
                frame 22 {
                  n3019 = property on="Samplingtime 2" class="DigNum (strict)"("Caption.Text"=w4050) -> ()  [unwired: 2 in, 2 out]
                }
                frame 23 {
                  "String 21" <- w4051
                }
                frame 24 {
                  n3020 = property on="Countdown" class="DigNum (strict)"("Caption.Text"=w4052) -> ()  [unwired: 2 in, 2 out]
                }
                frame 25 {
                  n3021 = property on="Countdown 2" class="DigNum (strict)"("Caption.Text"=w4053) -> ()  [unwired: 2 in, 2 out]
                }
                frame 26 {
                  n3022 = property on="Engage" class="Bool (strict)"("Boolean Text.Text"=w4054) -> ()  [unwired: 2 in, 2 out]
                }
                frame 27 {
                  n3023 = property on="Boolean  4" class="Bool (strict)"("Boolean Text.Text"=w4055) -> ()  [unwired: 2 in, 2 out]
                }
                frame 28 {
                  n3024 = property on="Test \nStatus" class="Bool (strict)"("Boolean Text.Text"=w4056) -> ()  [unwired: 2 in, 2 out]
                }
                frame 29 {
                }
                frame 30 {
                }
                frame 31 {
                }
                frame 32 {
                  n3025 = property on="RSTCOF" class="Bool"("Boolean Text.Text"=w4058) -> ()  [unwired: 2 in, 2 out]
                  n3026 = property on="RST FF" class="Bool"("Boolean Text.Text"=w4058) -> ()  [unwired: 2 in, 2 out]
                  n3027 = property on="RST TEMP" class="Bool"("Boolean Text.Text"=w4058) -> ()  [unwired: 2 in, 2 out]
                  n3028 = property on="RSTV1 3" class="Bool"("Boolean Text.Text"=w4058) -> ()  [unwired: 2 in, 2 out]
                  n3029 = property on="rstv2" class="Bool"("Boolean Text.Text"=w4058) -> ()  [unwired: 2 in, 2 out]
                  n3030 = property on="RSTV1 2" class="Bool"("Boolean Text.Text"=w4058) -> ()  [unwired: 2 in, 2 out]
                  n3031 = property on="RST CP" class="Bool"("Boolean Text.Text"=w4058) -> ()  [unwired: 2 in, 2 out]
                }
                frame 33 {
                  "S 61" <- w4059
                }
                frame 34 {
                  "String 23" <- w4060
                }
                frame 35 {
                  n3032 = property on="Rh Before" class="DigNum (strict)"("Caption.Text"=w4061) -> ()  [unwired: 2 in, 2 out]
                }
                frame 36 {
                  n3033 = Match Pattern(string=w4062, regular expression=",") -> (before substring=→"bs":string, after substring=→"as":string)  [unwired: 1 in, 2 out]
                  n3034 = property on="Rh After" class="DigNum (strict)"("Caption.Text"=w4062) -> ()  [unwired: 2 in, 2 out]
                }
                frame 37 {
                  n3035 = Match Pattern(string=w4071, regular expression=",") -> (before substring=w4070:string, after substring=w4069:string)  [unwired: 1 in, 2 out]
                  "bs" <- w4070
                  "as" <- w4069
                  n3036 = Concatenate Strings(w4070, w4069) -> (w4066:string)
                  n3037 = property on="Humidity before test 2" class="DigNum (strict)"("Caption.Text"=w4066) -> ()  [unwired: 2 in, 2 out]
                  n3038 = property on="Humidity before test" class="DigNum (strict)"("Caption.Text"=w4066) -> ()  [unwired: 2 in, 2 out]
                  n3039 = Concatenate Strings(w4066, "=" ("string")) -> (w4067:string)
                  n3040 = local write "S 38"(w4067) -> ()
                }
                frame 38 {
                  n3041 = Match Pattern(string=w4078, regular expression=",") -> (before substring=w4077:string, after substring=w4076:string)  [unwired: 1 in, 2 out]
                  "bs" <- w4077
                  "as" <- w4076
                  n3042 = Concatenate Strings(w4077, w4076) -> (w4073:string)
                  n3043 = property on="Humidity after test 2" class="DigNum (strict)"("Caption.Text"=w4073) -> ()  [unwired: 2 in, 2 out]
                  n3044 = Concatenate Strings(w4073, "=" ("string")) -> (w4075:string)
                  n3045 = property on="Humidity after test" class="DigNum (strict)"("Caption.Text"=w4073) -> ()  [unwired: 2 in, 2 out]
                  n3046 = local write "S 39"(w4075) -> ()
                }
                frame 39 {
                  n3047 = Match Pattern(string=w4085, regular expression=",") -> (before substring=w4084:string, after substring=w4083:string)  [unwired: 1 in, 2 out]
                  "bs" <- w4084
                  "as" <- w4083
                  n3048 = Concatenate Strings(w4084, w4083) -> (w4080:string)
                  n3049 = property on="Temperature before test 2" class="DigNum (strict)"("Caption.Text"=w4080) -> ()  [unwired: 2 in, 2 out]
                  n3050 = property on="Temperature before test" class="DigNum (strict)"("Caption.Text"=w4080) -> ()  [unwired: 2 in, 2 out]
                  n3051 = Concatenate Strings(w4080, "=" ("string")) -> (→"String 34":string)
                }
                frame 40 {
                  n3052 = Match Pattern(string=w4092, regular expression=",") -> (before substring=w4091:string, after substring=w4090:string)  [unwired: 1 in, 2 out]
                  "bs" <- w4091
                  "as" <- w4090
                  n3053 = Concatenate Strings(w4091, w4090) -> (w4087:string)
                  n3054 = property on="Temperature after test 2" class="DigNum (strict)"("Caption.Text"=w4087) -> ()  [unwired: 2 in, 2 out]
                  n3055 = Concatenate Strings(w4087, "=" ("string")) -> (→"String 35":string)
                  n3056 = property on="Temperature after test" class="DigNum (strict)"("Caption.Text"=w4087) -> ()  [unwired: 2 in, 2 out]
                }
                frame 41 {
                  n3057 = property on="AVP" class="DigNum (strict)"("Caption.Text"=w4096) -> ()  [unwired: 2 in, 2 out]
                  n3058 = property on="AVP 2" class="DigNum (strict)"("Caption.Text"=w4096) -> ()  [unwired: 2 in, 2 out]
                  n3059 = Concatenate Strings(w4096, "=" ("string")) -> (→"String 36":string)
                }
                frame 42 {
                  n3060 = property on="MWSD" class="DigNum (strict)"("Caption.Text"=w4099) -> ()  [unwired: 2 in, 2 out]
                  n3061 = property on="MWSD 2" class="DigNum (strict)"("Caption.Text"=w4099) -> ()  [unwired: 2 in, 2 out]
                  n3062 = Concatenate Strings(w4099, "=" ("string")) -> (→"String 37":string)
                }
                frame 43 {
                  n3063 = property on="HCF 2" class="DigNum (strict)"("Caption.Text"=w4102) -> ()  [unwired: 2 in, 2 out]
                  n3064 = property on="HCF" class="DigNum (strict)"("Caption.Text"=w4102) -> ()  [unwired: 2 in, 2 out]
                  n3065 = Concatenate Strings(w4102, "=" ("string")) -> (→"String 38":string)
                }
                frame 44 {
                  n3066 = Concatenate Strings(w4104, "=" ("string")) -> (→"String 39":string)
                  n3067 = property on="WS1.4 2" class="DigNum (strict)"("Caption.Text"=w4104) -> ()  [unwired: 2 in, 2 out]
                  n3068 = property on="WS1.4" class="DigNum (strict)"("Caption.Text"=w4104) -> ()  [unwired: 2 in, 2 out]
                }
                frame 45 {
                  n3069 = property on="Save Results" class="Bool (strict)"("Boolean Text.Text"=w4106) -> ()  [unwired: 2 in, 2 out]
                }
                frame 46 {
                  n3070 = local write "S 47"(w4107) -> ()
                }
                frame 47 {
                  n3071 = local write "S 48"(w4108) -> ()
                }
                frame 48 {
                  n3072 = local write "S 49"(w4109) -> ()
                }
                frame 49 {
                  n3073 = local write "S 50"(w4110) -> ()
                }
                frame 50 {
                  n3074 = local write "S 51"(w4111) -> ()
                }
                frame 51 {
                  n3075 = local write "S 52"(w4112) -> ()
                }
                frame 52 {
                  n3076 = local write "S 53"(w4113) -> ()
                }
                frame 53 {
                  n3077 = local write "S 54"(w4114) -> ()
                }
                frame 54 {
                  n3078 = local write "S 55"(w4115) -> ()
                }
                frame 55 {
                  n3079 = local write "S 56"(w4116) -> ()
                }
                frame 56 {
                  n3080 = local write "S 57"(w4117) -> ()
                }
                frame 57 {
                  n3081 = local write "S 58"(w4118) -> ()
                }
                frame 58 {
                  n3082 = local write "S 59"(w4119) -> ()
                }
                frame 59 {
                  n3083 = local write "S 60"(w4120) -> ()
                }
                frame 60 {
                  n3084 = local write "S 62"(w4121) -> ()
                }
                frame 61 {
                  n3085 = local write "S 63"(w4122) -> ()
                }
                frame 62 {
                  n3086 = local write "S 64"(w4123) -> ()
                }
                frame 63 {
                  n3087 = local write "S 65"(w4124) -> ()
                }
                frame 64 {
                  n3088 = local write "S 66"(w4125) -> ()
                }
                frame 65 {
                  n3089 = local write "S 67"(w4126) -> ()
                }
                frame 66 {
                  n3090 = local write "S 68"(w4127) -> ()
                }
                frame 67 {
                  n3091 = local write "S 69"(w4128) -> ()
                }
                frame 68 {
                  n3092 = local write "S 70"(w4129) -> ()
                }
                frame 69 {
                  n3093 = local write "S 71"(w4130) -> ()
                }
                frame 70 {
                  n3094 = local write "S 72"(w4131) -> ()
                }
                frame 71 {
                  n3095 = local write "S 73"(w4132) -> ()
                }
                frame 72 {
                  n3096 = local write "S 74"(w4133) -> ()
                }
                frame 73 {
                  n3097 = local write "S 75"(w4134) -> ()
                }
                frame 74 {
                  n3098 = local write "S 76"(w4135) -> ()
                }
                frame 75 {
                  n3099 = local write "S 77"(w4136) -> ()
                }
                frame 76 {
                  n3100 = local write "S 78"(w4137) -> ()
                }
                frame 77 {
                  n3101 = local write "S 79"(w4138) -> ()
                }
                frame 79 {
                  n3102 = property on="Sample Temperature ( °C )" class="XYGraph (strict)"("Y Scale.Name Label.Text"=w4139) -> ()  [unwired: 2 in, 2 out]
                }
                frame 80 {
                  n3103 = local write "S 81"(w4140) -> ()
                  n3104 = property on="Humidity ( %RH )" class="XYGraph (strict)"("Y Scale.Name Label.Text"=w4140) -> ()  [unwired: 2 in, 2 out]
                }
                frame 78 {
                  n3105 = property on="Air Temperature  ( °C )" class="XYGraph (strict)"("X Scale.Name Label.Text"=w4141) -> ()  [unwired: 2 in, 2 out]
                  n3106 = property on="Humidity ( %RH )" class="XYGraph (strict)"("X Scale.Name Label.Text"=w4141) -> ()  [unwired: 2 in, 2 out]
                  n3107 = property on="Sample Temperature ( °C )" class="XYGraph (strict)"("X Scale.Name Label.Text"=w4141) -> ()  [unwired: 2 in, 2 out]
                  n3108 = property on="Coefficient Of Friction" class="XYGraph (strict)"("X Scale.Name Label.Text"=w4141) -> ()  [unwired: 2 in, 2 out]
                }
                frame 81 {
                  n3109 = property on="Air Temperature  ( °C )" class="XYGraph (strict)"("Y Scale.Name Label.Text"=w4142) -> ()  [unwired: 2 in, 2 out]
                }
                frame 82 {
                  n3110 = local write "S 84"(w4143) -> ()
                }
                frame 83 {
                  n3111 = local write "S 85"(w4144) -> ()
                }
                frame 84 {
                  n3112 = local write "S 86"(w4145) -> ()
                }
                frame 85 {
                  n3113 = local write "S 87"(w4146) -> ()
                }
                frame 86 {
                  n3114 = local write "S 88"(w4147) -> ()
                }
                frame 87 {
                }
                frame 88 {
                  n3115 = local write "S 90"(w4149) -> ()
                }
                frame 89 {
                  n3116 = local write "S 91"(w4150) -> ()
                }
                frame 90 {
                  n3117 = local write "S 92"(w4151) -> ()
                }
                frame 91 {
                  n3118 = local write "S 93"(w4152) -> ()
                }
                frame 92 {
                  n3119 = local write "S 94"(w4153) -> ()
                }
                frame 93 {
                  n3120 = local write "S 95"(w4154) -> ()
                }
                frame 94 {
                  n3121 = local write "S 96"(w4155) -> ()
                }
                frame 95 {
                  n3122 = local write "S 97"(w4156) -> ()
                }
                frame 96 {
